vi "Add scale to image.vi"(5 "English Units? (metric)":bool, 6 "Color Box":u32(colorbox)=15664896, 7 "Show Scale (T)":bool=TRUE, 8 "error in":errorcluster, 9 "Scale name":string, 10 "Pixel Size (um)":dbl, 11 "Image In":T1) -> (0 "error out":errorcluster, 3 "Image Out":T1)   [LabVIEW 2012]
doc: "This Optionally adds a salbar as an overlay to an Image Buffer.\nThe pixel size in um is required."
uses:
  <vilib>/vision/Image Controls.llb/IMAQ Image.ctl
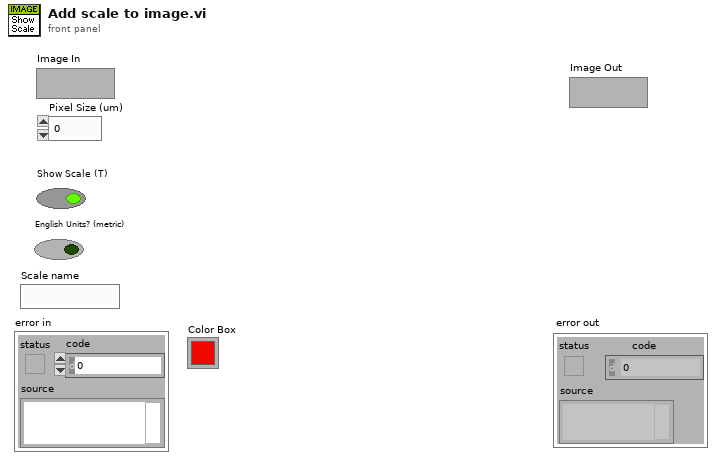
[diagram p1: front panel]
types:
  T1 = typedef "IMAQ Image.ctl" = refnum<image>
  T2 = cluster{"Desired Font (Application)":enum16{"User-specified Font", "Application Font", "System Font", "Dialog Font"}, "[User-specified Font]":cluster{"Font Name":string, "Size":i16, "Strikeout?":bool, "Italic?":bool, "Underline?":bool, "Outline?":bool, "Shadow?":bool, "Bold?":bool, "Rotation Angle":dbl}, "Horizontal Alignment":i16, "Vertical Alignment":i16}
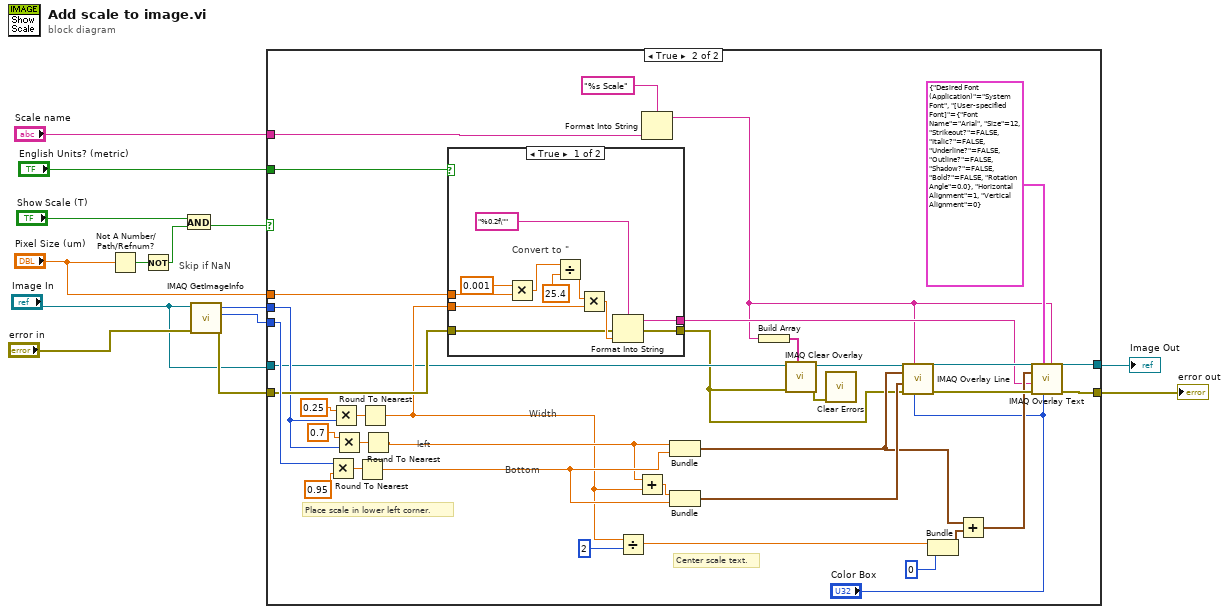
[diagram p0: block diagram]
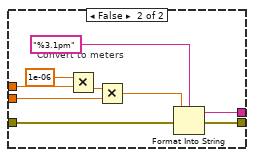
[diagram p3: hidden frame]
diagram:
  # "Skip if NaN"
  n1 = Not A Number/Path/Refnum?(number/path/refnum="Pixel Size (um)") -> (NaN/Path/Refnum?=w5:bool)
  n2 = Not(x=w5) -> (.not. x?=w4:bool)
  n3 = And(x="Show Scale (T)", y=w4) -> (x .and. y?=w3:bool)
  n4 = call "IMAQ GetImageInfo"("error in (no error)"="error in", "Image"="Image In") -> ("error out"=w10:errorcluster, "Y Resolution"=w11:i32, "X Resolution"=w12:i32)  [unwired: 7 out]
  n5 = case shown="True" w3 {
    tunnel: [w15 w50] -> w14
    tunnel: "Image In" -> [w16 w24]
    tunnel: w10 -> [w15 w32]
    tunnel: "Pixel Size (um)" -> [_ w33]
    tunnel: [w16 w39] -> w8
    tunnel: w12 -> [_ w28]
    tunnel: w11 -> [_ w34]
    tunnel: "English Units? (metric)" -> [_ w26]
    tunnel: "Scale name" -> [_ w19]
    frame False {
    }
    frame True {
      # "Bottom"
      # "left"
      # "Width"
      # "Center scale text."
      # "Place scale in lower left corner."
      n6 = Multiply(x=w34, y=0.95) -> (x*y=w36:dbl)
      n7 = Multiply(x=0.25, y=w28) -> (x*y=w37:dbl)
      n8 = Multiply(x=0.7, y=w28) -> (x*y=w31:dbl)
      n9 = Round To Nearest(number=w36) -> (nearest integer value=w35:dbl)
      n10 = Round To Nearest(number=w37) -> (nearest integer value=w27:dbl)
      n11 = Round To Nearest(number=w31) -> (nearest integer value=w29:dbl)
      n12 = case shown="True" w26 {
        tunnel: [w63 w72] -> w25
        tunnel: w33 -> [w61 w70]
        tunnel: w32 -> [w59 w67]
        tunnel: [w58 w66] -> w22
        tunnel: w27 -> [w57 w65]
        frame True {
          # "Convert to \""
          n13 = Multiply(x=0.001, y=w61) -> (x*y=w55:dbl)
          n14 = Divide(x=w55, y=25.4) -> (x/y=w56:dbl)
          n15 = Multiply(x=w56, y=w57) -> (x*y=w62:dbl)
          n16 = Format Into String(format string="%0.2f\"", error in=w59, w62) -> (resulting string=w63:string, error out=w58:errorcluster)  [unwired: 1 in]
        }
        frame False {
          # "Convert to meters"
          n17 = Multiply(x=1e-06, y=w70) -> (x*y=w68:dbl)
          n18 = Multiply(x=w68, y=w65) -> (x*y=w71:dbl)
          n19 = Format Into String(format string="%3.1pm", error in=w67, w71) -> (resulting string=w72:string, error out=w66:errorcluster)  [unwired: 1 in]
        }
      }
      n20 = Divide(x=w27, y=2) -> (x/y=w40:dbl)
      n21 = Add(x=w29, y=w27) -> (x+y=w46:dbl)
      n22 = Format Into String(format string="%s Scale", w19) -> (resulting string=w20:string)  [unwired: 2 in, 1 out]
      n23 = Bundle(w29, w35) -> (w43:cluster{dbl, dbl})  [unwired: 1 out]
      n24 = Bundle(w46, w35) -> (w49:cluster{dbl, dbl})  [unwired: 1 out]
      n25 = Build Array(w20) -> (w18:string[])
      n26 = call "IMAQ Clear Overlay"("Groups"=w18, "error in (no error)"=w22, "Image"=w24) -> ("error out"=w17:errorcluster, "Image Out"=w23:T1)  [unwired: 7 out]
      n27 = call <vilib>:"Clear Errors.vi"("error in (no error)"=w17) -> ()  [unwired: 7 out]
      n28 = call "IMAQ Overlay Line"("Color"="Color Box", "Group"=w20, "error in (no error)"=w22, "End Point"=w49, "Start Point"=w43, "Image"=w23) -> ("error out"=w51:errorcluster, "Image Out"=w52:T1)  [unwired: 4 out]
      n29 = Bundle(w40, "y"=0) -> (w44:cluster{dbl, "y":i32})  [unwired: 1 out]
      n30 = Add(x=w43, y=w44) -> (x+y=w42:cluster{dbl, dbl})
      n31 = call "IMAQ Overlay Text"("Group"=w20, "Text Color (black)"="Color Box", "Font, Size & Style"=T2 {"Desired Font (Application)"=enum."System Font", "[User-specified Font]"={"Font Name"="Arial", "Size"=12, "Strikeout?"=FALSE, "Italic?"=FALSE, "Underline?"=FALSE, "Outline?"=FALSE, "Shadow?"=FALSE, "Bold?"=FALSE, "Rotation Angle"=0.0}, "Horizontal Alignment"=1, "Vertical Alignment"=0}, "error in (no error)"=w51, "String"=w25, "Origin"=w42, "Image"=w52) -> ("error out"=w50:errorcluster, "Image Out"=w39:T1)  [unwired: 1 in, 2 out]
    }
  }
  "error out" <- w14
  "Image Out" <- w8
